vi "Send.vi"(7 "VolatusAPI":refnum<class "VolatusAPI.lvclass">, 10 "Value":dbl, 11 "Numeric Command in":refnum<class "Numeric Command.lvclass">) -> (0 "error out":errorcluster)   [LabVIEW 2023, in "Volatus.lvlib" / "Numeric Command.lvclass"]
uses:
  Numeric Command.lvclass
  VolatusAPI/VolatusAPI.lvclass
  Numeric Command.lvclass/Numeric Command.ctl
  messages/CmdAnalog/Class/Msg.lvclass/Msg.ctl
  VolatusAPI/VolatusAPI.lvclass/VolatusAPI.ctl
  MessageQ/MessageQ.lvclass/MessageQ.ctl
  messages/CmdAnalog/Class/Msg.lvclass
  lv-vecto/Vecto/TCPMessageService/Send Message.vi
  <vilib>/Utility/error.llb/Error Cluster From Error Code.vi
  lv-protoc/LV-Proto/Message/Message.lvclass
  MessageQ/MessageQ.lvclass
  messages/CmdAnalogMultiple/Class/Msg.lvclass
  messages/CmdAnalogMultiple/CmdAnalogMultiple.lvlib
  C:/dev/volatus/mts-volatus-super/libs/lv-volatus/messages/CmdAnalogMultiple/Class/Msg.lvclass
  C:/dev/volatus/mts-volatus-super/libs/lv-protoc/LV-Proto/Message/Message.lvclass
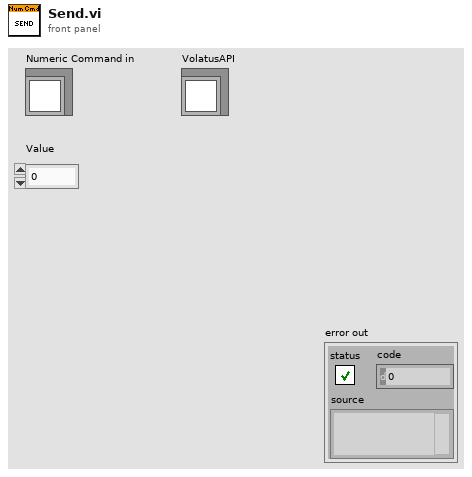
[diagram p1: front panel]
types:
  T1 = typedef "CmdAnalog.lvlib/Data.ctl" = cluster{"channel":string, "value":dbl}
  T2 = typedef "CmdAnalogMultiple.lvlib/Data.ctl" = cluster{"values":T1[]}
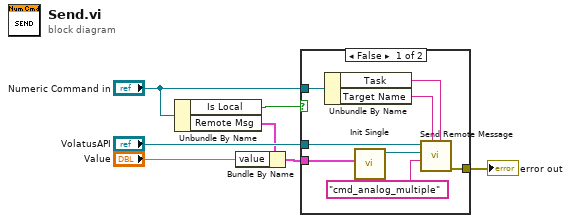
[diagram p0: block diagram]
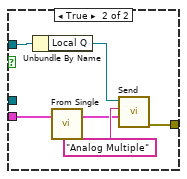
[diagram p2: hidden frame]
diagram:
  n1 = Unbundle By Name("Numeric Command in") -> ("Is Local"=w7:bool, "Remote Msg"=w5:T1)
  n2 = Bundle By Name(cluster=w5, "value"="Value") -> (w3:T1)
  n3 = case shown="False" w7 {
    tunnel: "VolatusAPI" -> [w15 _]
    tunnel: w3 -> [w14 w18]
    tunnel: "Numeric Command in" -> [w11 w21]
    tunnel: [w8 w17] -> w1
    frame False {
      n4 = Unbundle By Name(w11) -> ("Task"=w9:string, "Target Name"=w10:string)
      n5 = call "Init Single.vi"("value"=w14) -> ("Msg out"=w13:refnum<class "Msg.lvclass">)  [unwired: 10 in]
      n6 = call "Send Remote Message.vi"("Target Task (None)"=w9, "Target Name"=w10, "Message Type"="cmd_analog_multiple", "Message"=w13, "VolatusAPI in"=w15) -> ("error out"=w8:errorcluster)  [unwired: 5 in, 1 out]
    }
    frame True {
      n7 = Unbundle By Name(w21) -> ("Local Q"=w20:refnum<class "MessageQ.lvclass">)
      n8 = call "From Single.vi"("CmdAnalog"=w18) -> ("CmdAnalogMultiple"=w16:T2)  [unwired: 6 in]
      n9 = call "Send.vi"("Data"=w16, "ID"="Analog Multiple", "MessageQ in"=w20) -> ("error out"=w17:errorcluster)  [unwired: 7 in, 1 out]
    }
  }
  "error out" <- w1
